vi "WriteLogWithTimestamp.vi"(8 "error in (no error)":errorcluster, 10 "Punktnummer":string, 11 "Byte Stream File in":refnum<file>) -> (0 "error out":errorcluster, 3 "Byte Stream File out":refnum<file>)   [LabVIEW 2017]
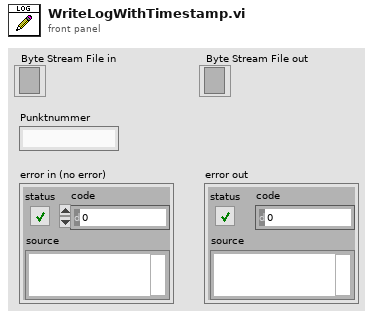
[diagram p1: front panel]
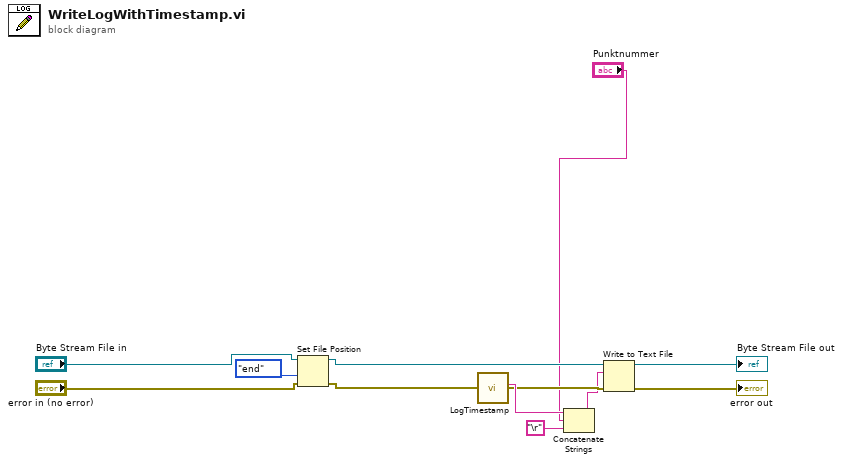
[diagram p0: block diagram]
diagram:
  n1 = Set File Position(refnum="Byte Stream File in", from (0:start)=enum16{"start", "end", "current"}."end", error in="error in (no error)") -> (refnum out=w11:refnum<file>, error out=w9:errorcluster)  [unwired: 1 in]
  n2 = call "LogTimestamp.vi"() -> ("Log Timestamp"=w10:string)  [unwired: 9 in, 1 out]
  n3 = Concatenate Strings(w10, "Punktnummer", "\r") -> (w5:string)
  n4 = Write to Text File(file (use dialog)=w11, text=w5, error in=w9) -> (refnum out=→"Byte Stream File out":refnum<file>, error out=→"error out":errorcluster)  [unwired: 1 in, 1 out]
